vi "Config ODX Path.vi"(8 "error in (no error)":errorcluster, 11 "Parttype":T1) -> (0 "error out":errorcluster)   [LabVIEW 2014]
uses:
  typedefs/parttype.ctl
  <vilib>/Utility/config.llb/Read Key (Path).vi
  <vilib>/Utility/config.llb/Write Key (Path).vi
  <vilib>/Utility/config.llb/NI_LVConfig.lvlib
panel:
  in  "Cancel":bool
  out "Current Path":path
  in  "Save":bool
  in  "New Path":path
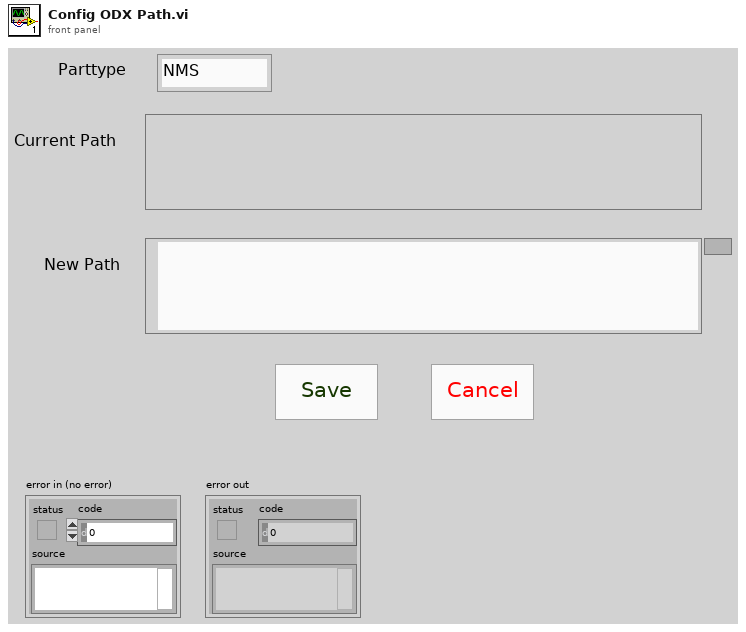
[diagram p1: front panel]
types:
  T1 = typedef "parttype.ctl" = enum16{"NMS", "B-SUV"}
  T2 = typedef "NI_LVConfig.lvlib/Config Data RefNum.ctl" = refnum<k1>
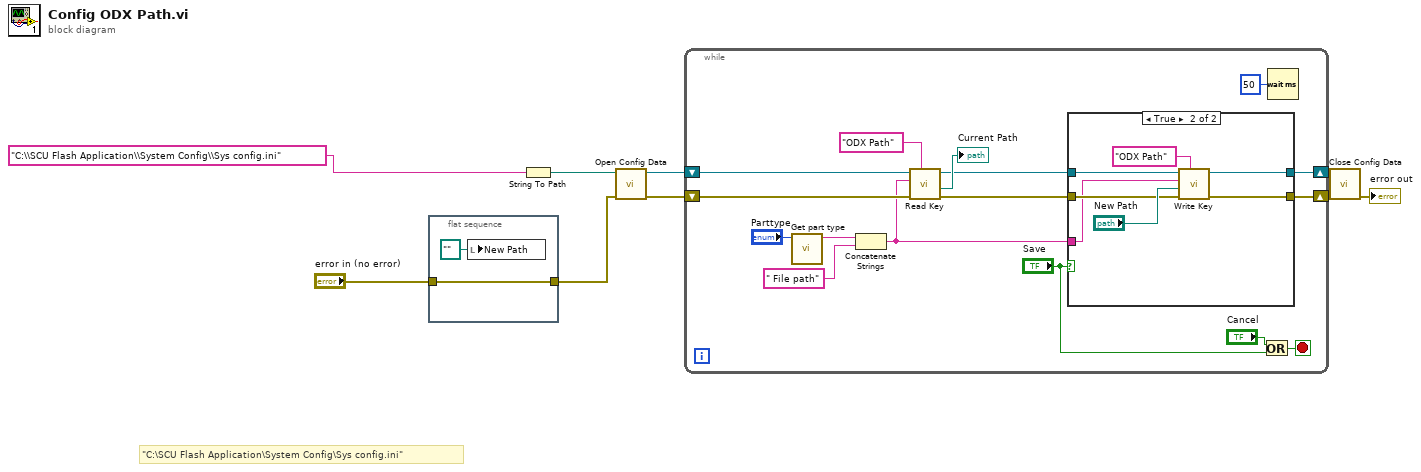
[diagram p0: block diagram]
diagram:
  # "\"C:\\SCU Flash Application\\System Config\\Sys config.ini\""
  n1 = flat-sequence {
    tunnel: "error in (no error)" -> [w10]
    tunnel: [w10] -> w4
    frame #0 {
      n2 = local write "New Path"(path "" ("New Path")) -> ()
    }
  }
  n3 = String To Path(string="C:\\SCU Flash Application\\System Config\\Sys config.ini" ("name or relative path")) -> (path=w9:path)
  n4 = call <vilib>:"Open Config Data.vi"("error in (no error)"=w4, "configuration file path"=w9) -> ("error out"=w2:errorcluster, "refnum"=w3:T2)  [unwired: 7 in, 1 out]
  n5 = while {
    shift-right: [w26] -> w7
    shift-left: w3 -> [w16]
    shift-right: [w25] -> w6
    shift-left: w2 -> [w15]
    stop <- w24 stop-if-true
    n6 = call "Get part type.vi"("Enum"="Parttype") -> ("Parttype"=w19:string)  [unwired: 10 in]
    n7 = Concatenate Strings(w19, " File path" ("string")) -> (w12:string)
    n8 = call-poly <vilib>:"Read Key.vi"("section"="ODX Path", "error in (no error)"=w15, "key"=w12, "refnum"=w16) -> ("error out"=w14:errorcluster, "value"=→"Current Path":path, "refnum out"=w13:T2)  [unwired: 4 in, 1 out]
    n9 = case shown="True" "Save" {
      tunnel: w13 -> [w29 w36]
      tunnel: [w29 w33] -> w26
      tunnel: [w28 w32] -> w25
      tunnel: w14 -> [w28 w31]
      tunnel: w12 -> [_ w30]
      frame False {
      }
      frame True {
        n10 = call-poly <vilib>:"Write Key.vi"("section"="ODX Path", "error in (no error)"=w31, "value"="New Path", "key"=w30, "refnum"=w36) -> ("error out"=w32:errorcluster, "refnum out"=w33:T2)  [unwired: 4 in, 1 out]
      }
    }
    n11 = Or(x="Cancel", y="Save") -> (x .or. y?=w24:bool)
    n12 = Wait (ms)(milliseconds to wait=u32 50) -> ()  [unwired: 1 out]
  }
  n13 = call <vilib>:"Close Config Data.vi"("error in (no error)"=w6, "refnum"=w7) -> ("error out"=→"error out":errorcluster)  [unwired: 8 in, 1 out]
